vi "Get Geo Codes.vi"(8 "error in (no error)":errorcluster, 9 "Country":T1=enum."Germany", 10 "City Name":string, 11 "Geocoding in":refnum<class "Geocoding.lvclass">) -> (0 "error out":errorcluster, 3 "Geocoding out":refnum<class "Geocoding.lvclass">)   [LabVIEW 2025, in "Geocoding Actor.lvlib" / "Geocoding.lvclass"]
uses:
  Geocoding.lvclass
  C:/Program Files (x86)/National Instruments/LabVIEW 2025/vi.lib/ActorFramework/Actor/Actor.lvclass
  Country.ctl
  <vilib>/ActorFramework/Actor/Actor.lvclass/Actor.ctl
  Geocoding.lvclass/Geocoding.ctl
  UI/UI Messages/Read Geo Coding Results Msg/Read Geo Coding Results Msg.lvclass/Read Geo Coding Results Msg.ctl
  <vilib>/ActorFramework/Message Enqueuer/Message Enqueuer.lvclass/Message Enqueuer.ctl
  <vilib>/ActorFramework/Message Enqueuer/Enqueue.vi
  UI/UI Messages/Read Geo Coding Results Msg/Read Geo Coding Results Msg.lvclass
  C:/Program Files (x86)/National Instruments/LabVIEW 2025/vi.lib/ActorFramework/Message/Message.lvclass
  <vilib>/ActorFramework/Message Priority Queue/Priority Enqueue.vi
  UI Launcher/UI Launcher.lvlib
  <vilib>/ActorFramework/Actor/Actor.lvclass
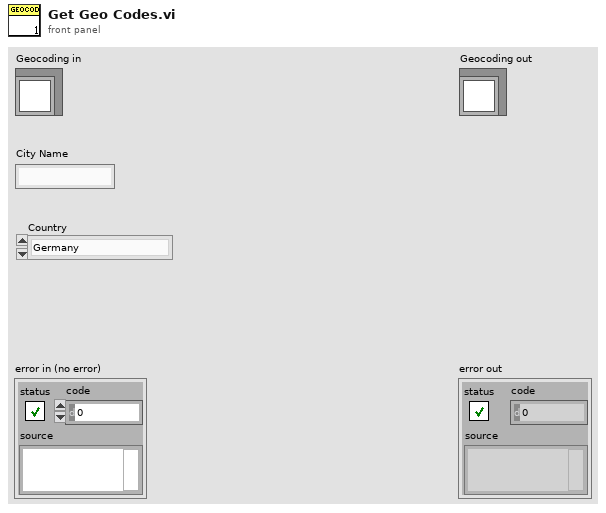
[diagram p1: front panel]
types:
  T1 = typedef "Geocoding Actor.lvlib/Geocoding.lvclass/Country.ctl" = enum16{"Austria", "Germany", "Switzerland"}
  T2 = cluster{"id":i32, "name":string, "latitude":dbl, "longitude":dbl, "elevation":dbl, "feature_code":string, "country_code":string, "timezone":string, "population":i32, "postcodes":string[], "admin1":string, "admin2":string, "admin3":string, "admin4":string, "admin1_id":i32, "admin2_id":i32, "admin3_id":i32, "admin4_id":i32}[]
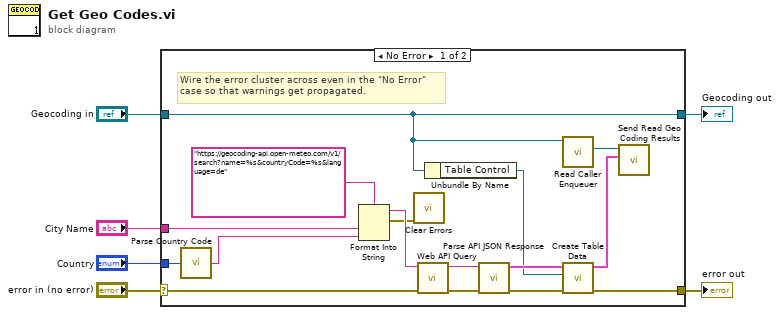
[diagram p0: block diagram]
diagram:
  n1 = case shown="No Error" "error in (no error)" {
    selector: "error in (no error)" -> [w20 w24]
    tunnel: [w11 w24] -> w5
    tunnel: [w8 w23] -> w3
    tunnel: "Geocoding in" -> [w8 w23]
    tunnel: "City Name" -> [w18 _]
    tunnel: "Country" -> [w17 _]
    frame No Error {
      # "Wire the error cluster across even in the \"No Error\"\ncase so that warnings get propagated."
      n2 = call "Parse Country Code.vi"("Country"=w17) -> ("Country Code"=w16:string)  [unwired: 4 in]
      n3 = Format Into String(format string="https://geocoding-api.open-meteo.com/v1/search?name=%s&countryCode=%s&language=de" ("url"), w18, w16) -> (resulting string=w15:string, error out=w14:errorcluster)  [unwired: 2 in]
      n4 = call <vilib>:"Clear Errors.vi"("error in (no error)"=w14) -> ()  [unwired: 5 in, 2 out]
      n5 = call "Web API Query.vi"("error in (no error)"=w20, "url"=w15) -> ("error out"=w21:errorcluster, "API Response"=w22:string)  [unwired: 8 in]
      n6 = Unbundle By Name(w8) -> ("Table Control"=w7:refnum<vi>)
      n7 = call "Parse API JSON Response.vi"("error in"=w21, "API Response"=w22) -> ("error out"=w12:errorcluster, "Results"=w10:T2)  [unwired: 8 in]
      n8 = call <vilib>:"Read Caller Enqueuer.vi"("Actor"=w8) -> ("Caller Enqueuer"=w13:refnum<class "Message Enqueuer.lvclass">)  [unwired: 10 in]
      n9 = call "Create Table Data.vi"("error in (no error)"=w12, "Table Control"=w7, "Results"=w10) -> ("error out"=w11:errorcluster, "Results out"=w9:T2)  [unwired: 7 in]
      n10 = call "Send Read Geo Coding Results.vi"("Geo Code Results"=w9, "Message Enqueuer"=w13) -> ()  [unwired: 8 in, 2 out]
    }
    frame Error {
    }
  }
  "error out" <- w5
  "Geocoding out" <- w3
